vi "ProviderShell.vi"(7 "MAL":T1, 8 "error in (no error)":errorcluster, 10 "Configuration":cluster{"A":dbl, "b":dbl}, 11 "Related HAL Devices":cluster{"HAL 1":T2}) -> (0 "error out":errorcluster, 2 "Result":dbl)   [LabVIEW 2019]
uses:
  MAL/lv-APT-MAL/MAL-Interface/Classes/MAL-Prototype/Typedef/Def-RelatedHALDevice.ctl
  MAL/lv-APT-MAL/MAL-Interface/Classes/MAL-Prototype/Typedef/Def-MALInformation.ctl
  e9bc0481-d5ec-4a79-8865-eb3ae7f53980.vi
  1a1087cd-0cbc-4370-a44a-3f340b268824.vi
  <vilib>/Utility/error.llb/Clear Errors.vi
  _support/fpMgr/fpMgr.lvclass
  MAL/lv-APT-MAL/MAL-Interface/Classes/MAL-Prototype/MAL-Prototype.lvclass
panel:
  out "Matched":bool
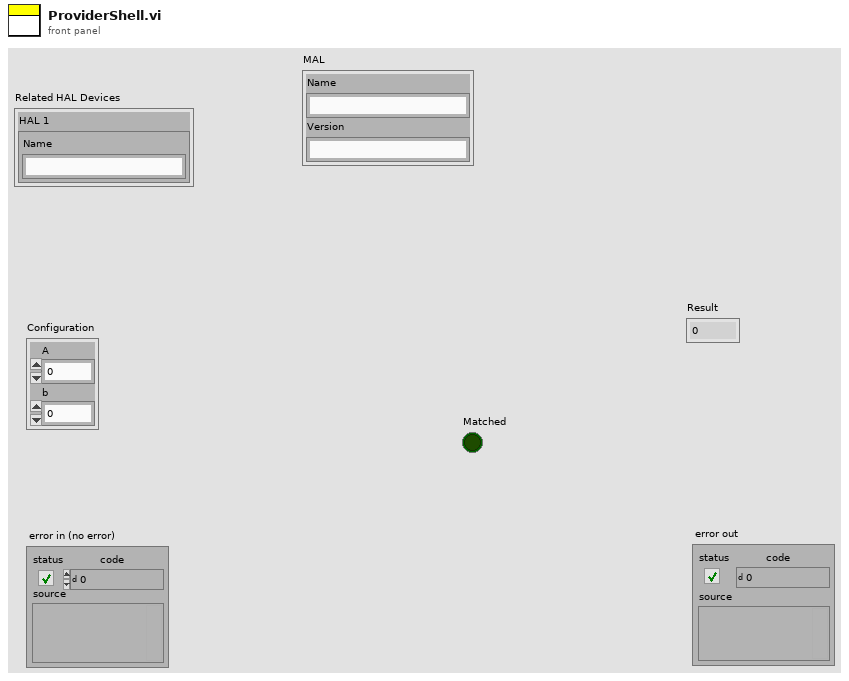
[diagram p1: front panel]
types:
  T1 = typedef "MAL-Interface.lvlib/MAL-Prototype.lvclass/Def-MALInformation.ctl" = cluster{"Name":string, "Version":string}
  T2 = typedef "MAL-Interface.lvlib/MAL-Prototype.lvclass/Def-RelatedHALDevice.ctl" = cluster{"Name":string}
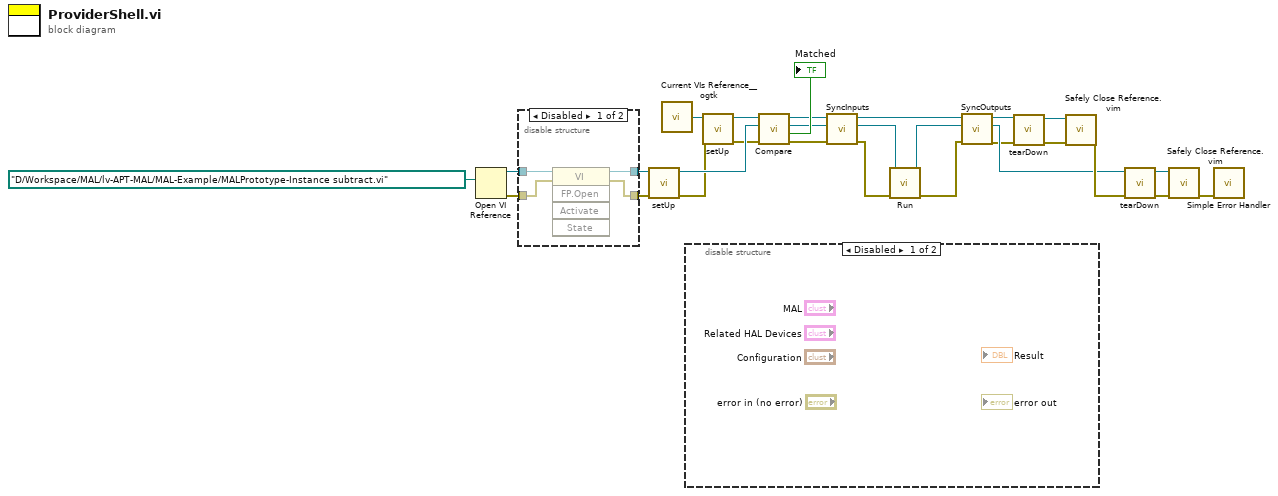
[diagram p0: block diagram]
diagram:
  n1 = Open VI Reference(vi path=path "D:/Workspace/MAL/lv-APT-MAL/MAL-Example/MALPrototype-Instance subtract.vi") -> (vi reference=w27:refnum<vi>, error out=w3:errorcluster)  [unwired: 5 in]
  n2 = disable-structure shown="Disabled" {
    disable-tunnel: w27 -> [w32 w34]
    disable-tunnel: [w31 w34] -> w4
    disable-tunnel: w3 -> [w30 w33]
    disable-tunnel: [w29 w33] -> w2
    frame Disabled {
      n3 = invoke class="VI" method="FP.Open"(reference=w32, error in=w30) -> (reference out=w31:refnum<vi>, error out=w29:errorcluster)  [unwired: 3 in, 3 out]
    }
    frame Enabled {
    }
  }
  n4 = call "setUp.vi"("error in (no error)"=w2, "VI in"=w4) -> ("error out"=w17:errorcluster, "fpMgr out"=w25:refnum<class "fpMgr.lvclass">)  [unwired: 8 in]
  n5 = call <userlib>:"Current VIs Reference__ogtk.vi"() -> ("Current VI's reference"=w16:refnum<vi>)  [unwired: 5 in]
  n6 = disable-structure shown="Disabled" {
    frame Disabled {
    }
    frame Enabled {
    }
  }
  n7 = call "setUp.vi"("error in (no error)"=w17, "VI in"=w16) -> ("error out"=w24:errorcluster, "fpMgr out"=w26:refnum<class "fpMgr.lvclass">)  [unwired: 8 in]
  n8 = call "Compare.vi"("error in (no error)"=w24, "fpMgr in"=w25, "Shell in"=w26) -> ("error out"=w7:errorcluster, "Matched"=→"Matched":bool, "fpMgr out"=w12:refnum<class "fpMgr.lvclass">, "Shell out"=w15:refnum<class "fpMgr.lvclass">)  [unwired: 5 in]
  n9 = call "SyncInputs.vi"("error in (no error)"=w7, "fpMgr in"=w12, "Shell in"=w15) -> ("error out"=w6:errorcluster, "fpMgr out"=w11:refnum<class "fpMgr.lvclass">, "Shell out"=w14:refnum<class "fpMgr.lvclass">)  [unwired: 6 in]
  n10 = call "Run.vi"("error in (no error)"=w6, "fpMgr in"=w11) -> ("error out"=w5:errorcluster, "fpMgr out"=w10:refnum<class "fpMgr.lvclass">)  [unwired: 8 in]
  n11 = call "SyncOutputs.vi"("error in (no error)"=w5, "fpMgr in"=w10, "Shell in"=w14) -> ("error out"=w8:errorcluster, "fpMgr out"=w9:refnum<class "fpMgr.lvclass">, "Shell out"=w13:refnum<class "fpMgr.lvclass">)  [unwired: 6 in]
  n12 = call "tearDown.vi"("error in (no error)"=w8, "fpMgr in"=w13) -> ("error out"=w22:errorcluster, "VI"=w23:refnum<vi>)  [unwired: 8 in]
  n13 = call "Safely Close Reference.vim"("error in (no error)"=w22, "LVClassLibrary in"=w23) -> ("error out"=w21:errorcluster)  [unwired: 9 in]
  n14 = call "tearDown.vi"("error in (no error)"=w21, "fpMgr in"=w9) -> ("error out"=w19:errorcluster, "VI"=w20:refnum<vi>)  [unwired: 8 in]
  n15 = call "Safely Close Reference.vim"("error in (no error)"=w19, "LVClassLibrary in"=w20) -> ("error out"=w1:errorcluster)  [unwired: 9 in]
  n16 = call <vilib>:"Simple Error Handler.vi"("error in (no error)"=w1) -> ()  [unwired: 4 in, 5 out]
